vi "Read.vi"(11 "GroupValue in":refnum<class "GroupAbstractValue.lvclass">) -> (2 "Group":refnum<class "Group.lvclass">)   [LabVIEW 2020, in "Vecto.lvlib" / "GroupAbstractValue.lvclass"]
uses:
  GroupAbstractValue.lvclass
  Group/Group.lvclass
  GroupAbstractValue.lvclass/GroupAbstractValue.ctl
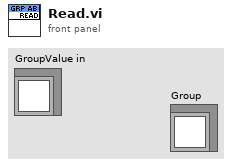
[diagram p1: front panel]
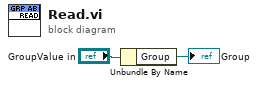
[diagram p0: block diagram]
diagram:
  n1 = Unbundle By Name("GroupValue in") -> ("Group"=→"Group":refnum<class "Group.lvclass">)
